vi "Get_Setup_Initial_Positions.vi"(1 "Setup Filename":string) -> (0 "Initial Offsets":sgl[](array[numeric]))   [LabVIEW 2022 SP3]
uses:
  File/Setup_Filetype.ctl
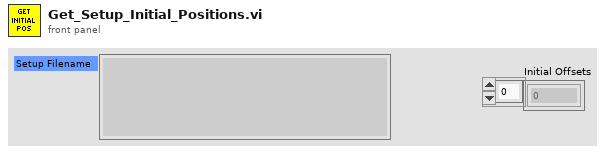
[diagram p1: front panel]
types:
  T1 = typedef "Setup_Filetype.ctl" = enum16{"Measurement Setups", "Calibration Setups", "General", "Results File Plotter Setups", "Speed Calib Tweaks"}
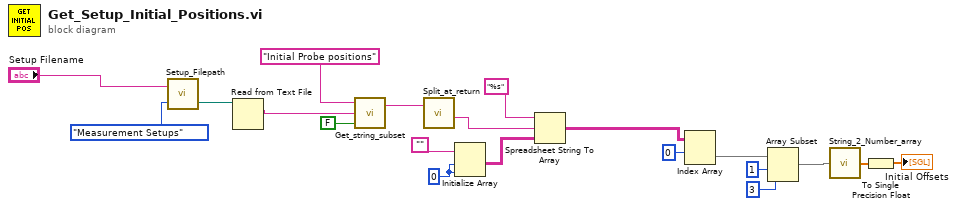
[diagram p0: block diagram]
diagram:
  w14 = 0 ("Dimension Size")
  n1 = call "Setup_Filepath.vi"("Setup File Type"=Setup_Filetype."Measurement Setups", "Filename in"="Setup Filename") -> ("Filename Out"=w19:path)  [unwired: 1 out]
  n2 = Read from Text File(file (use dialog)=w19) -> (text=w16:string)  [unwired: 3 in, 3 out]
  n3 = call "Get_string_subset.vi"("Show Dialog?"=FALSE, "String to split"=w16, "File Label"="Initial Probe positions") -> ("Output string"=w10:string)  [unwired: 1 in, 1 out]
  n4 = call "Split_at_return.vi"("String"=w10) -> ("after substring"=w11:string)  [unwired: 1 in, 3 out]
  n5 = Initialize Array("", w14, w14) -> (w15:string[][])
  n6 = Spreadsheet String To Array(format string="%s", spreadsheet string=w11, array type (2D Dbl)=w15) -> (array=w5:string[][])  [unwired: 1 out]
  n7 = Index Array(array=w5, index (row)=0) -> (element=w9:string[])  [unwired: 1 in]
  n8 = Array Subset(array=w9, index=1, length=3) -> (w8:string[])
  n9 = call "String_2_Number_array.vi"("Input String"=w8) -> ("Values"=w3:dbl[])
  n10 = To Single Precision Float(number=w3) -> (single precision float=→"Initial Offsets":sgl[])
